vi "Create_Data_Cluster.vi"() -> (3 "Cluster":T1)   [LabVIEW 2016]
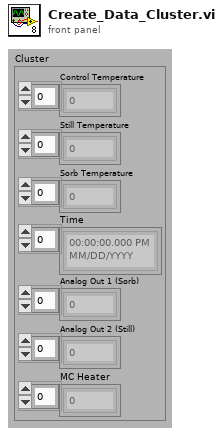
[diagram p1: front panel]
types:
  T1 = cluster{"Control Temperature":dbl[], "Still Temperature":dbl[], "Sorb Temperature":dbl[], "Time":timestamp[], "Analog Out 1 (Sorb)":dbl[], "Analog Out 2 (Still)":dbl[], "MC Heater":dbl[]}
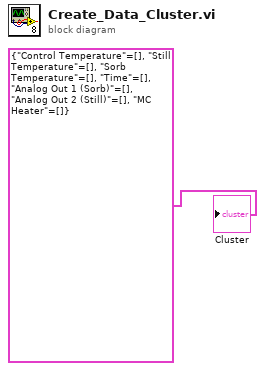
[diagram p0: block diagram]
diagram:
  "Cluster" <- T1 {"Control Temperature"=[], "Still Temperature"=[], "Sorb Temperature"=[], "Time"=[], "Analog Out 1 (Sorb)"=[], "Analog Out 2 (Still)"=[], "MC Heater"=[]}
